vi "subExportVIContent.vi"(6 "CodeSchema":string, 8 "error in (no error)":errorcluster, 9 "Expand?":bool, 10 "Add virtual folders?":bool, 11 "ILabVIEWItem in":refnum<class "ILabVIEWItem.lvclass">) -> (0 "error out":errorcluster, 1 "Links":T1, 2 "Nodes":T1, 3 "ILabVIEWItem out":refnum<class "ILabVIEWItem.lvclass">)   [LabVIEW 2020, in "DefaultExtensions.lvlib" / "CGrapherDGML.lvclass"]
uses:
  CGrapherDGML.lvclass
  obj/Addons/LabVIEWObjectInterfaces.lvlibp/LabVIEWObjectInterfaces/ILabVIEWItem/ILabVIEWItem.lvclass
  obj/Addons/LabVIEWItem.lvlibp/LabVIEWItem/CLabVIEWItem/ConnectionSet.ctl
  obj/Addons/LabVIEWItem.lvlibp/LabVIEWItem/CLabVIEWItem/CLabVIEWItem.lvclass
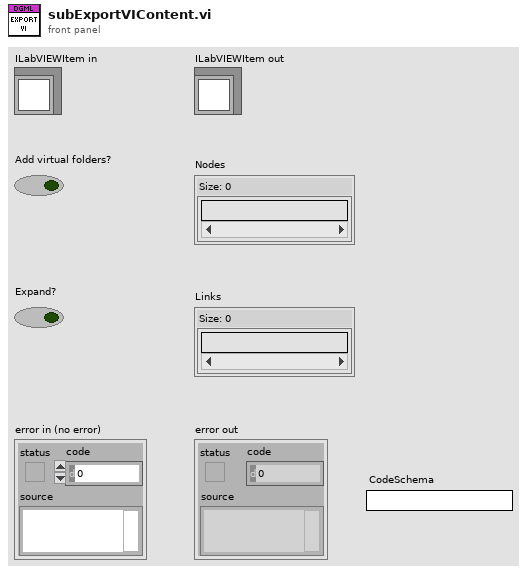
[diagram p1: front panel]
types:
  T1 = typedef "LabVIEWItem.lvlibp/CLabVIEWItem.lvclass/ConnectionSet.ctl" = set{string}
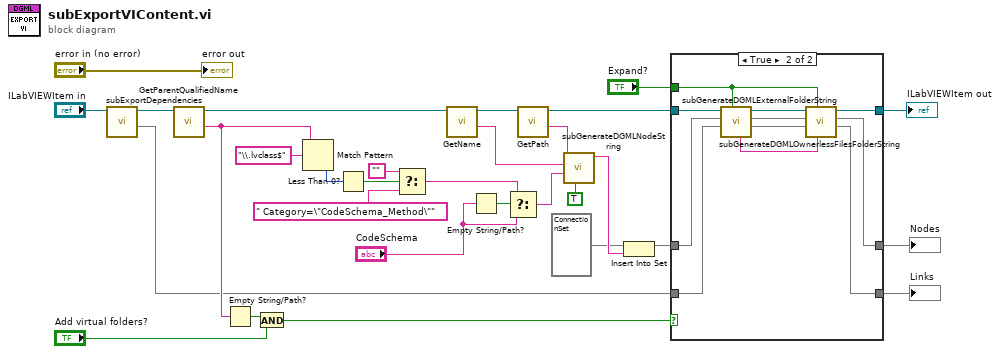
[diagram p0: block diagram]
diagram:
  n1 = call "subExportDependencies.vi"("ILabVIEWItem in"="ILabVIEWItem in") -> ("Links"=w16:T1, "ILabVIEWItem out"=w28:refnum<class "ILabVIEWItem.lvclass">)  [unwired: 8 in, 1 out]
  n2 = call-dynamic "GetParentQualifiedName.vi"("ILabVIEWItem in"=w28) -> ("Name"=w19:string, "ILabVIEWItem out"=w27:refnum<class "ILabVIEWItem.lvclass">)  [unwired: 8 in, 1 out]
  n3 = Empty String/Path?(string/path=w19) -> (empty?=w13:bool)
  n4 = And(x=w13, y="Add virtual folders?") -> (x .and. y?=w11:bool)
  n5 = Match Pattern(string=w19, regular expression="\\.lvclass$") -> (offset past match=w25:i32)  [unwired: 1 in, 3 out]
  n6 = Less Than 0?(x=w25) -> (x < 0?=w24:bool)
  n7 = Select(t="", s=w24, f=" Category=\"CodeSchema_Method\"") -> (s? t:f=w21:string)
  n8 = call-dynamic "GetName.vi"("ILabVIEWItem in"=w27) -> ("Name"=w10:string, "ILabVIEWItem out"=w2:refnum<class "ILabVIEWItem.lvclass">)  [unwired: 8 in, 1 out]
  n9 = Empty String/Path?(string/path="CodeSchema") -> (empty?=w20:bool)
  n10 = Select(t=w21, s=w20, f="CodeSchema") -> (s? t:f=w9:string)
  n11 = call-dynamic "GetPath.vi"("ILabVIEWItem in"=w2) -> ("Path"=w7:string, "ILabVIEWItem out"=w6:refnum<class "ILabVIEWItem.lvclass">)  [unwired: 8 in, 1 out]
  n12 = call "subGenerateDGMLNodeString.vi"("Container empty?"=TRUE, "Code schema"=w9, "Label"=w10, "Id"=w7) -> ("Node string"=w8:string)  [unwired: 7 in]
  n13 = Insert Into Set(10:w8, 11:T1 {} ("Links")) -> (3:w18:T1)  [unwired: 1 out]
  n14 = case shown="True" w11 {
    tunnel: w16 -> [w32 w42]
    tunnel: [w32 w35] -> w15
    tunnel: w18 -> [w33 w43]
    tunnel: [w33 w34] -> w17
    tunnel: "Expand?" -> [_ w40]
    tunnel: w6 -> [w31 w44]
    tunnel: [w31 w36] -> w5
    frame False {
    }
    frame True {
      n15 = call "subGenerateDGMLOwnerlessFilesFolderString.vi"("Expand?"=w40, "Links in"=w42, "Nodes in"=w43, "ILabVIEWItem in"=w44) -> ("Links"=w38:T1, "Nodes"=w39:T1, "ILabVIEWItem out"=w41:refnum<class "ILabVIEWItem.lvclass">, "Path"=w37:string)  [unwired: 3 in, 1 out]
      n16 = call "subGenerateDGMLExternalFolderString.vi"("Path in"=w37, "Expand?"=w40, "Links in"=w38, "Nodes in"=w39, "ILabVIEWItem in"=w41) -> ("Links"=w35:T1, "Nodes"=w34:T1, "ILabVIEWItem out"=w36:refnum<class "ILabVIEWItem.lvclass">)  [unwired: 3 in, 1 out]
    }
  }
  "ILabVIEWItem out" <- w5
  "Nodes" <- w17
  "Links" <- w15
  "error out" <- "error in (no error)"
